vi "Draw Preview.vi"(5 "BG Color":u32(colorbox)=15724527, 7 "Box Color":u32(colorbox)=15724527, 8 "Border (px) [4]":i16=4, 9 "Height (px) [40]":i16=40, 10 "Width (px) [64]":i16=64, 11 "Plot Bounds":T1[](array[typedef]) {"Plot Bounds (%)"."Bottom (%)" format="%.2f"; "Plot Bounds (%)"."Top (%)" format="%.2f"; "Plot Bounds (%)"."Right (%)" format="%.2f"; "Plot Bounds (%)"."Left (%)" format="%.2f"}) -> (3 "Preview Pict":picture)   [LabVIEW 2021, in "MultiRocketPlotPanel.lvclass"]
uses:
  Classes/MultiPlotPanel/MultiRocketPlotPanel.lvclass
  Window Position and plot number.ctl
  Window Position.ctl
panel:
  out "Array":T3(array[cluster])
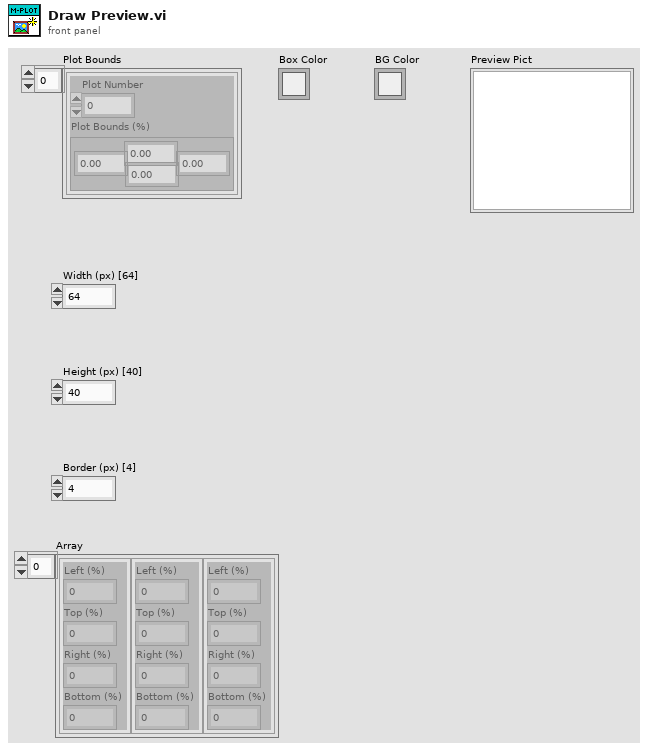
[diagram p1: front panel]
types:
  T1 = typedef "MultiRocketPlotPanel.lvclass/Window Position and plot number.ctl" = cluster{"Plot Number":i32, "Plot Bounds (%)":T2}
  T2 = typedef "MultiRocketPlotPanel.lvclass/Window Position.ctl" = cluster{"Left (%)":dbl, "Top (%)":dbl, "Right (%)":dbl, "Bottom (%)":dbl}
  T3 = cluster{"Left (%)":i16, "Top (%)":i16, "Right (%)":i16, "Bottom (%)":i16}[]
  T4 = cluster{"left":i16, "top":i16, "right":i16, "bottom":i16}
  T5 = cluster{"Width":i16, "Style":enum32{"Solid", "Dash", "Dot", "DashDot", "DashDotDot"}}
  T6 = cluster{"Left (%)":i16, "Top (%)":i16, "Right (%)":i16, "Bottom (%)":i16}
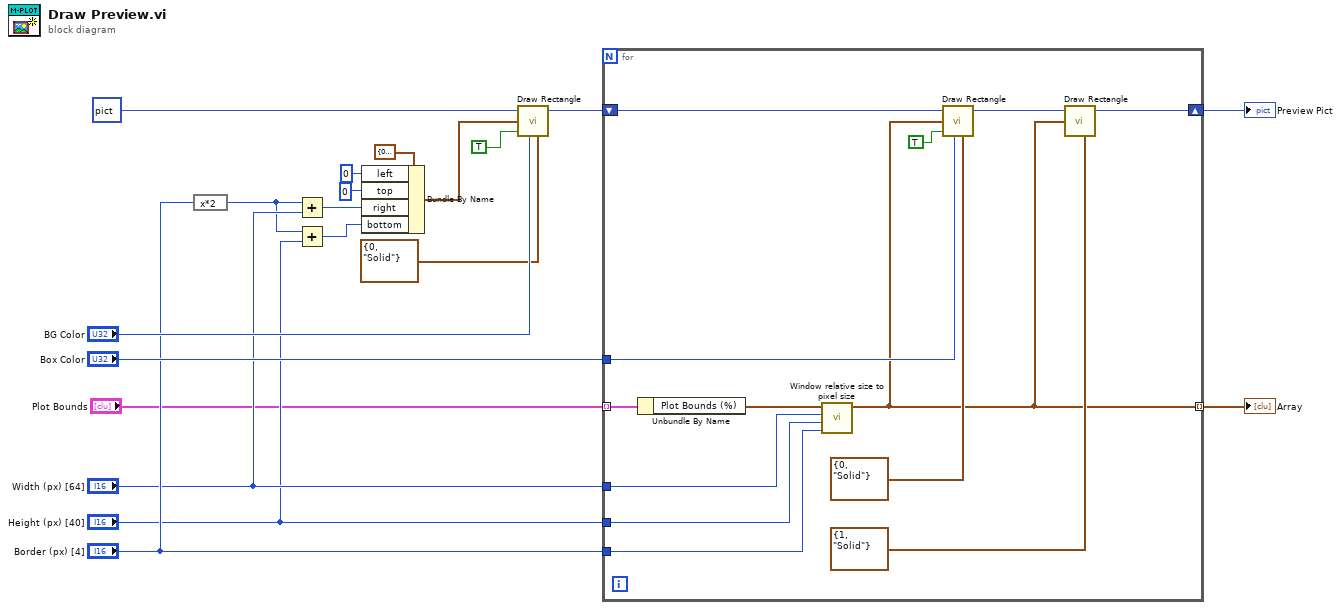
[diagram p0: block diagram]
diagram:
  n1 = expression code="x*2"("Border (px) [4]") -> (w7:i16)
  n2 = Add(x=w7, y="Width (px) [64]") -> (x+y=w4:i16)
  n3 = Add(x=w7, y="Height (px) [40]") -> (x+y=w3:i16)
  n4 = Bundle By Name(cluster=T4 {"left"=0, "top"=0, "right"=0, "bottom"=0} ("rect"), "left"=i16 0, "top"=i16 0 ("right"), "right"=w4, "bottom"=w3) -> (w2:T4)
  n5 = call <vilib>:"Draw Rectangle.vi"("picture"=picture data[5B], "rect"=w2, "fill?(F)"=TRUE, "color(black)"="BG Color", "pen"=T5 {"Width"=0, "Style"=enum."Solid"}) -> ("new picture"=w15:picture)  [unwired: 4 in]
  n6 = for {
    tunnel: "Plot Bounds" -> [w21] mode=indexing
    shift-right: [w26] -> w18
    shift-left: w15 -> [w32]
    tunnel: "Box Color" -> [w30]
    tunnel: [w25] -> w17 mode=indexing
    tunnel: "Width (px) [64]" -> [w24]
    tunnel: "Height (px) [40]" -> [w23]
    tunnel: "Border (px) [4]" -> [w22]
    n7 = Unbundle By Name(w21) -> ("Plot Bounds (%)"=w20:T2)
    n8 = call "Window relative size to pixel size.vi"("Border (px)"=w22, "Height (px)"=w23, "Width (px)"=w24, "Window Relative Size (%)"=w20) -> ("16bit integer"=w25:T6)  [unwired: 7 in]
    n9 = call <vilib>:"Draw Rectangle.vi"("picture"=w32, "rect"=w25, "fill?(F)"=TRUE, "color(black)"=w30, "pen"=T5 {"Width"=0, "Style"=enum."Solid"}) -> ("new picture"=w28:picture)  [unwired: 4 in]
    n10 = call <vilib>:"Draw Rectangle.vi"("picture"=w28, "rect"=w25, "pen"=T5 {"Width"=1, "Style"=enum."Solid"}) -> ("new picture"=w26:picture)  [unwired: 6 in]
  }
  "Preview Pict" <- w18
  "Array" <- w17
